vi "Control Auto Exposure.vi"(8 "error in":errorcluster) -> (0 "error out":errorcluster, 1 "Control Error":bool, 2 "Auto Exposure Time":bool)   [LabVIEW 2009]
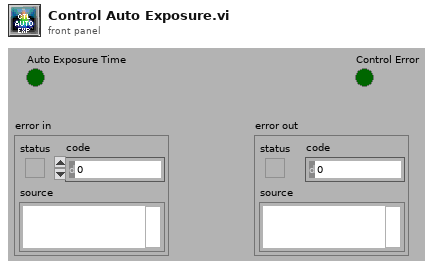
[diagram p1: front panel]
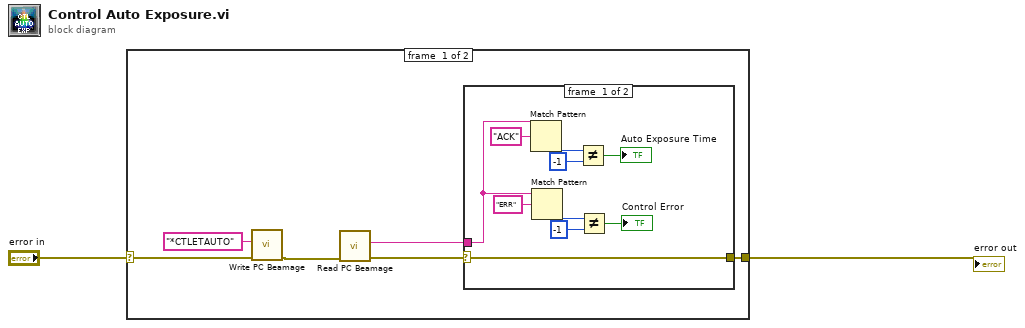
[diagram p0: block diagram]
diagram:
  n1 = case shown="No Error" "error in" {
    selector: "error in" -> [w7 w20]
    tunnel: [w3 w20] -> w1
    frame #0 {
      n2 = call "Write PC Beamage.vi"("error in"=w7, "command"="*CTLETAUTO") -> ("error out"=w6:errorcluster)  [unwired: 9 in]
      n3 = call "Read PC Beamage.vi"("error in"=w6) -> ("error out"=w5:errorcluster, "Reply"=w4:string)  [unwired: 9 in]
      n4 = case shown="No Error" w5 {
        selector: w5 -> [w9 w19]
        tunnel: w4 -> [w10 _]
        tunnel: [w9 w19] -> w3
        frame #0 {
          n5 = Match Pattern(string=w10, regular expression="ACK") -> (offset past match=w17:i32)  [unwired: 1 in, 3 out]
          n6 = Match Pattern(string=w10, regular expression="ERR") -> (offset past match=w13:i32)  [unwired: 1 in, 3 out]
          n7 = Not Equal?(x=w17, y=-1) -> (x != y?=→"Auto Exposure Time":bool)
          n8 = Not Equal?(x=w13, y=-1) -> (x != y?=→"Control Error":bool)
        }
        frame #1 {
        }
      }
    }
    frame #1 {
    }
  }
  "error out" <- w1
